vi "Copy_Proj_Data.vi"(8 "error in (no error)":errorcluster, 9 "IB_Destination.lvclass":refnum<class "IB_Destination.lvclass">, 10 "IB_Tree_Item_Proj in":refnum<class "IB_Tree_Item_Proj.lvclass">, 11 "IB_Source_Build in":refnum<class "IB_Source_Build.lvclass">) -> (0 "error out":errorcluster, 3 "IB_Source_Build out":refnum<class "IB_Source_Build.lvclass">)   [LabVIEW 2020, in "IB_Source_Build.lvclass"]
uses:
  <vilib>/AppBuilder/IB_Classes/Source/Container/Build/IB_Source_Build.lvclass
  <vilib>/AppBuilder/IB_Classes/Source/Container/Build/IB_Source_Build.lvclass/IB_Source_Build.ctl
  <vilib>/AppBuilder/IB_Classes/Source/Container/IB_Source_Container.lvclass
  <vilib>/AppBuilder/IB_Classes/Tree_Item_Proj_Build/IB_Tree_Item_Proj_Build.lvclass
  <vilib>/AppBuilder/IB_Classes/Tree_Item_Proj/IB_Tree_Item_Proj.lvclass
  <vilib>/AppBuilder/IB_Classes/Destination/IB_Destination.lvclass
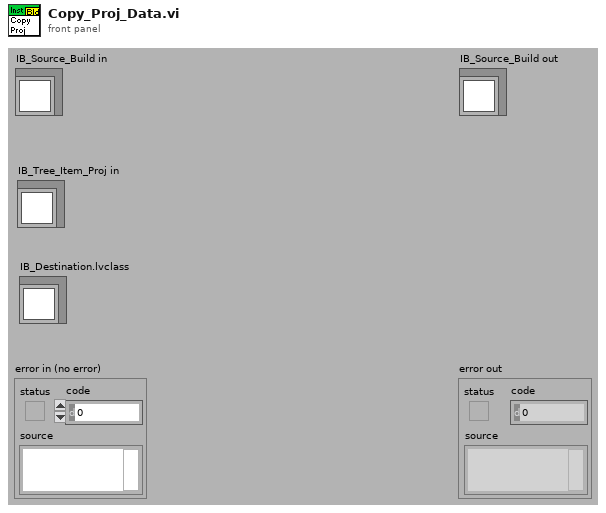
[diagram p1: front panel]
types:
  T1 = typedef "AB_Dependency.ctl" = cluster{"path":path, "delimited name":string, "type":T2}
  T2 = typedef "NI_FileType.lvlib/LVFileType.ctl" = enum32{"Invalid file", "Unknown type", "Instrument", "Control", "Polymorphic VI", "Project", "Library", "LVClass", "XControl", "XNode", "Shared library", ".NET assembly", "ActiveX interface", "CIN", "Run-time menu", "Palette menu", "Help file", "LLB", "XNode Edit Dependency", "Class Private Data Control", "Statechart", "MathScript .m file", "Ladder Diagram", "LVLibp", "XNode Build Dependency"}
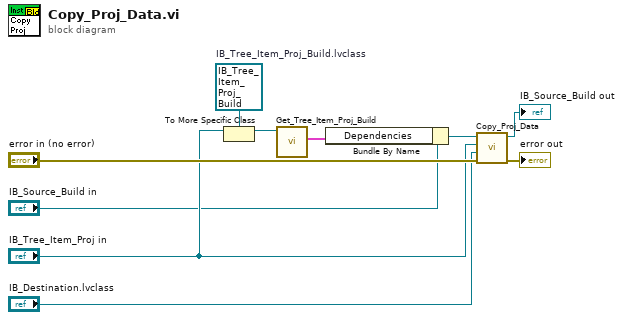
[diagram p0: block diagram]
diagram:
  w6 = refnum<class "IB_Tree_Item_Proj_Build.lvclass"> refnum  # IB_Tree_Item_Proj_Build.lvclass
  n1 = To More Specific Class(target class=w6, reference="IB_Tree_Item_Proj in") -> (specific class reference=w4:refnum<class "IB_Tree_Item_Proj_Build.lvclass">)  [unwired: 1 in, 1 out]
  n2 = call <vilib>:"Get_Tree_Item_Proj_Build.vi"("IB_Tree_Item_Proj_Build in"=w4) -> ("Dependencies"=w1:T1[])  [unwired: 8 in, 2 out]
  n3 = Bundle By Name(cluster="IB_Source_Build in", "Dependencies"=w1) -> (w2:refnum<class "IB_Source_Build.lvclass">)
  n4 = call-parent "Copy_Proj_Data.vi"("error in (no error)"="error in (no error)", "IB_Destination.lvclass"="IB_Destination.lvclass", "IB_Tree_Item_Proj in"="IB_Tree_Item_Proj in", "IB_Source_Container in"=w2) -> ("error out"=→"error out":errorcluster, "IB_Source_Container out"=→"IB_Source_Build out":refnum<class "IB_Source_Build.lvclass">)  [unwired: 6 in]
